vi "soundwave_generator_v02_offline_player.vi"() -> ()   [LabVIEW 2019]
uses:
  <vilib>/sound2/lvsound2.llb/Sound Data Format.ctl
  <vilib>/sound2/lvsound2.llb/Sampling Mode.ctl
  <vilib>/sound2/lvsound2.llb/Sound File Read Open.vi
  <vilib>/sound2/lvsound2.llb/Sound File Read (DBL).vi
  <vilib>/sound2/lvsound2.llb/Sound Output Set Volume (Single).vi
  <vilib>/sound2/lvsound2.llb/Sound Output Write (DBL).vi
  <vilib>/Waveform/WDTOps.llb/WDT Waveform Duration DBL.vi
panel:
  in  "Path":path=path "D:/Scuola Superiore Sant'Anna/Neuro-Robotic Touch Laboratory - PhD Marian Statache - PhD Marian Statache/03 - HW & SW/Sound Psychophysical Protocol v3/sound_samples/2sec_352-00_396-00_412-50_440-00_469-33_495-00_528-00/2sec_AAd_440-00_469-33.wav"
  in  "volume 1":dbl(slide)=50.0 scale=0.0..100.0
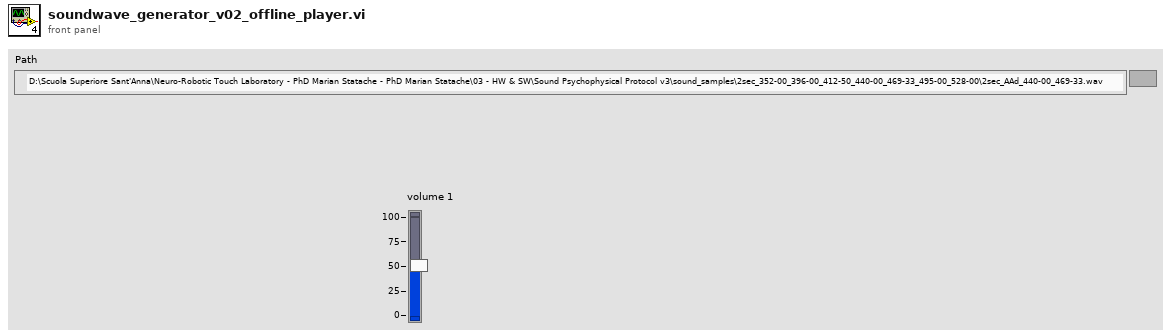
[diagram p1: front panel]
types:
  T1 = typedef "Sampling Mode.ctl" = i32
  T2 = typedef "Sound Data Format.ctl" = cluster{"sample rate (S/s)":dbl, "number of channels":i32, "bits per sample":i32}
  T3 = typedef "Sound File Refnum.ctl" = refnum<file>
  T4 = typedef "Sound Output Task ID.ctl" = u32
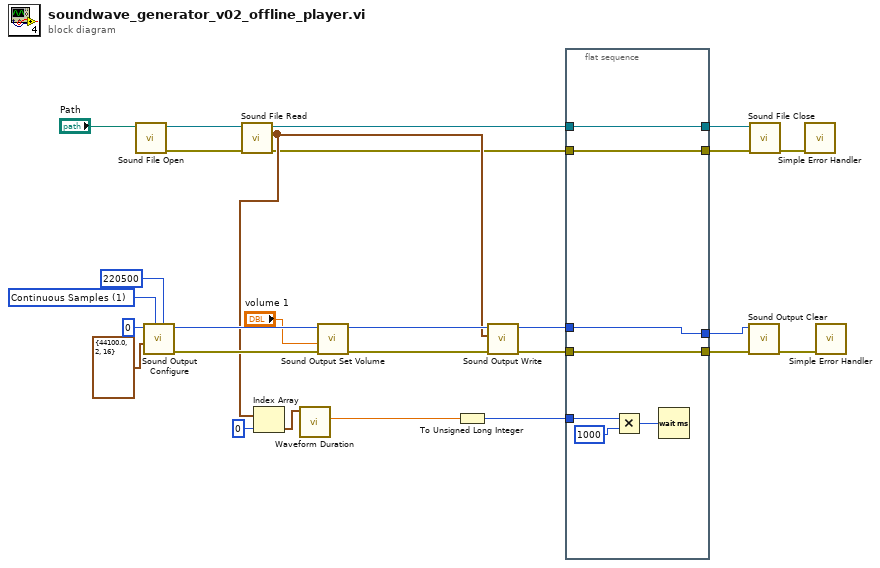
[diagram p0: block diagram]
diagram:
  w22 = T1 1 items=["Finite Samples", "Continuous Samples"] ("sample mode")
  n1 = call-poly <vilib>:"Sound File Open.vi"("path"="Path") -> ("error out"=w16:errorcluster, "sound file refnum"=w17:T3)  [unwired: 9 in]
  n2 = call <vilib>:"Sound Output Configure.vi"("number of samples/ch"=220500, "sample mode"=w22, "sound format"=T2 {"sample rate (S/s)"=44100.0, "number of channels"=2, "bits per sample"=16}, "device ID"=u32 0) -> ("error out"=w24:errorcluster, "task ID"=w23:T4)  [unwired: 6 in]
  n3 = call-poly <vilib>:"Sound File Read.vi"("error in (no error)"=w16, "sound file refnum"=w17) -> ("error out"=w7:errorcluster, "data"=w12:waveform(dbl)[], "sound file refnum out"=w8:T3)  [unwired: 5 in, 2 out]
  n4 = Index Array(array=w12, index=0) -> (element=w10:waveform(dbl))
  n5 = call-poly <vilib>:"Waveform Duration.vi"("waveform in"=w10) -> ("duration"=w1:dbl)  [unwired: 8 in, 2 out]
  n6 = call-poly <vilib>:"Sound Output Set Volume.vi"("error in (no error)"=w24, "volume"="volume 1", "task ID"=w23) -> ("error out"=w13:errorcluster, "task ID out"=w14:T4)  [unwired: 7 in]
  n7 = To Unsigned Long Integer(number=w1) -> (unsigned 32bit integer=w25:u32)
  n8 = call-poly <vilib>:"Sound Output Write.vi"("error in (no error)"=w13, "data"=w12, "task ID"=w14) -> ("error out"=w3:errorcluster, "task ID out"=w4:T4)  [unwired: 7 in]
  n9 = flat-sequence {
    tunnel: w25 -> [w34]
    tunnel: [w31] -> w9
    tunnel: w8 -> [w31]
    tunnel: w7 -> [w30]
    tunnel: [w30] -> w6
    tunnel: [w29] -> w5
    tunnel: w4 -> [w29]
    tunnel: w3 -> [w28]
    tunnel: [w28] -> w2
    frame #0 {
      n10 = Multiply(x=w34, y=u32 1000) -> (x*y=w32:u32)
      n11 = Wait (ms)(milliseconds to wait=w32) -> ()  [unwired: 1 out]
    }
  }
  n12 = call <vilib>:"Sound Output Clear.vi"("error in (no error)"=w2, "task ID"=w5) -> ("error out"=w27:errorcluster)  [unwired: 9 in]
  n13 = call <vilib>:"Sound File Close.vi"("error in (no error)"=w6, "sound file refnum"=w9) -> ("error out"=w26:errorcluster)  [unwired: 9 in]
  n14 = call <vilib>:"Simple Error Handler.vi"("error in (no error)"=w26) -> ()  [unwired: 4 in, 5 out]
  n15 = call <vilib>:"Simple Error Handler.vi"("error in (no error)"=w27) -> ()  [unwired: 4 in, 5 out]
